vi "CMD_UNLOADSTAMP.vi"(6 "Gantry in":refnum<class "Gantry.lvclass">, 8 "error in (no error)":errorcluster, 10 "Arguments":string[](array[string]), 11 "gScript Interpreter in":refnum<class "gScript Interpreter.lvclass">) -> (0 "error out":errorcluster, 3 "gScript Interpreter out":refnum<class "gScript Interpreter.lvclass">, 4 "Gantry out":refnum<class "Gantry.lvclass">)   [LabVIEW 2017, in "gScript Interpreter.lvclass"]
uses:
  gScript Interpreter.lvclass
  Shared Components/Gantry Class/Gantry.lvclass
  Shared Components/FlexWorktable/FlexWorktable.lvclass
  Shared Components/Vec3d Class/Vec3d.lvclass
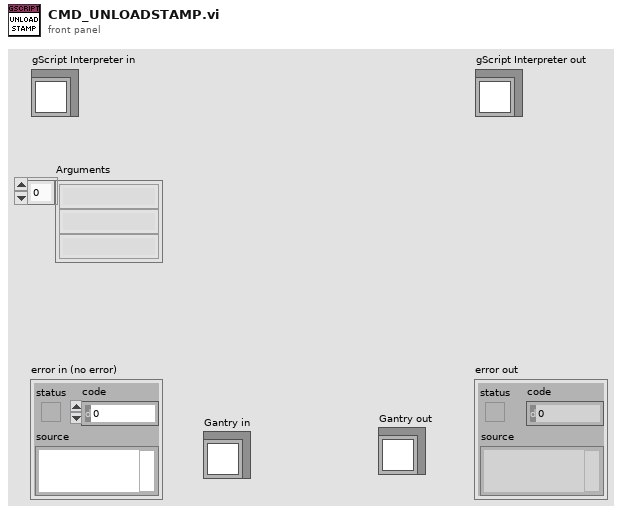
[diagram p1: front panel]
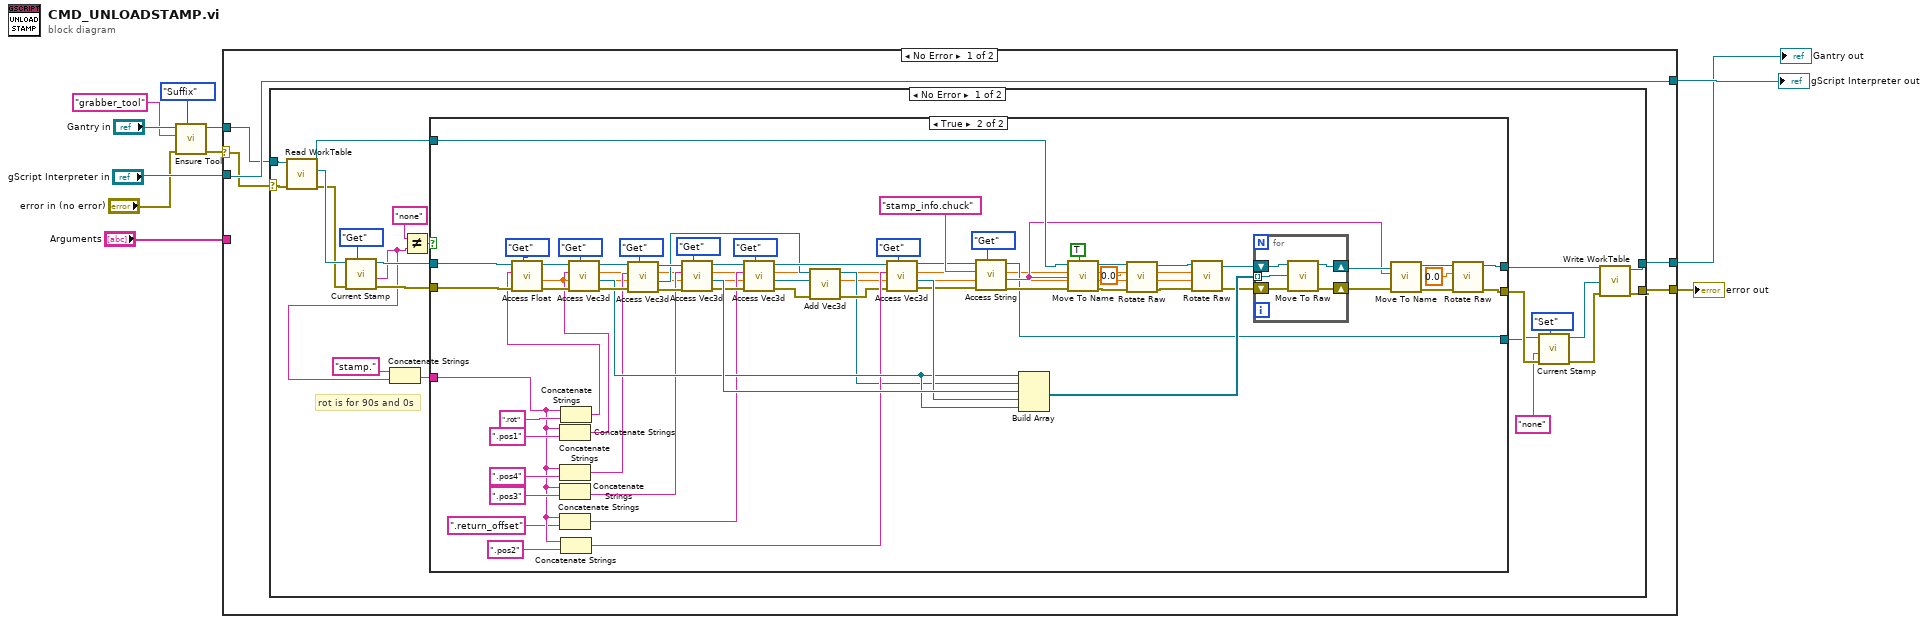
[diagram p0: block diagram]
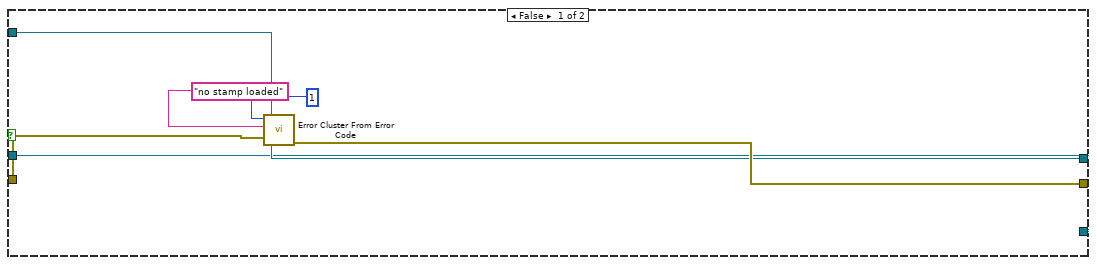
[diagram p2: hidden frame]
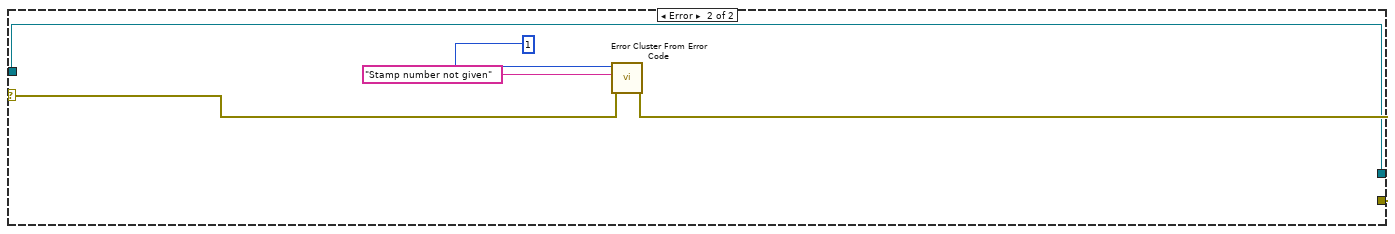
[diagram p3: hidden frame]
diagram:
  n1 = call "Ensure Tool.vi"("Match Type"=enum16{"Full", "Suffix"}."Suffix", "error in (no error)"="error in (no error)", "Tool Name"="grabber_tool", "Gantry in"="Gantry in") -> ("error out"=w3:errorcluster, "Gantry out"=w6:refnum<class "Gantry.lvclass">)  [unwired: 6 in]
  n2 = case shown="No Error" w3 {
    selector: w3 -> [w13 w120]
    tunnel: [w16 w120] -> w11
    tunnel: [w14 w119] -> w9
    tunnel: "gScript Interpreter in" -> [w14 w119]
    tunnel: w6 -> [w12 w118]
    tunnel: [w15 w118] -> w8
    tunnel: "Arguments" -> [_ _]
    frame No Error {
      n3 = case shown="No Error" w13 {
        selector: w13 -> [w38 w114]
        tunnel: [w29 w115] -> w16
        tunnel: w12 -> [w37 w113]
        tunnel: [w28 w113] -> w15
        frame No Error {
          # "rot is for 90s and 0s"
          n4 = call-dynamic "Read WorkTable.vi"("error in"=w38, "Gantry Class in"=w37) -> ("error out"=w23:errorcluster, "Worktable"=w36:refnum<class "FlexWorktable.lvclass">, "Gantry Class out"=w27:refnum<class "Gantry.lvclass">)  [unwired: 7 in]
          n5 = call "Current Stamp.vi"("Get/Set"=enum16{"Get", "Set"}."Get", "error in (no error)"=w23, "FlexWorktable in"=w36) -> ("error out"=w34:errorcluster, "Current Stamp"=w19:string, "FlexWorktable out"=w26:refnum<class "FlexWorktable.lvclass">)  [unwired: 6 in]
          n6 = Concatenate Strings("stamp.", w19) -> (w21:string)
          n7 = Not Equal?(x="none", y=w19) -> (x != y?=w20:bool)
          n8 = case shown="True" w20 {
            tunnel: [w41 w57] -> w30
            tunnel: w34 -> [w42 w91]
            tunnel: w27 -> [w40 w76]
            tunnel: [w40 w56] -> w25
            tunnel: w26 -> [w39 w105]
            tunnel: [w39 w69] -> w24
            tunnel: w21 -> [_ w46]
            frame False {
              n9 = call <vilib>:"Error Cluster From Error Code.vi"("error in (no error)"=w42, "error message (\"\")"="no stamp loaded" ("error message (\"\")"), "error code (0)"=1) -> ("error out"=w41:errorcluster)  [unwired: 6 in]
            }
            frame True {
              n10 = Concatenate Strings(w46, ".pos1" ("string")) -> (w83:string)
              n11 = Concatenate Strings(w46, ".pos4" ("string")) -> (w82:string)
              n12 = Concatenate Strings(w46, ".pos3" ("string")) -> (w81:string)
              n13 = Concatenate Strings(w46, ".return_offset" ("Key")) -> (w62:string)
              n14 = Concatenate Strings(w46, ".rot" ("string")) -> (w79:string)
              n15 = call-dynamic "Access Float.vi"("Get/Set"=enum16{"Get", "Set"}."Get", "error in (no error)"=w91, "Key"=w79, "FlexWorktable in"=w105) -> ("error out"=w107:errorcluster, "Value out"=w52:dbl, "FlexWorktable out"=w106:refnum<class "FlexWorktable.lvclass">)  [unwired: 5 in]
              n16 = Concatenate Strings(w46, ".pos2" ("string")) -> (w80:string)
              n17 = call-dynamic "Access Vec3d.vi"("Get/Set"=enum16{"Get", "Set"}."Get", "error in (no error)"=w107, "Key"=w83, "FlexWorktable in"=w106) -> ("error out"=w104:errorcluster, "Value out"=w89:refnum<class "Vec3d.lvclass">, "FlexWorktable out"=w103:refnum<class "FlexWorktable.lvclass">)  [unwired: 5 in]
              n18 = call-dynamic "Access Vec3d.vi"("Get/Set"=enum16{"Get", "Set"}."Get", "error in (no error)"=w104, "Key"=w82, "FlexWorktable in"=w103) -> ("error out"=w102:errorcluster, "Value out"=w59:refnum<class "Vec3d.lvclass">, "FlexWorktable out"=w101:refnum<class "FlexWorktable.lvclass">)  [unwired: 5 in]
              n19 = call-dynamic "Access Vec3d.vi"("Get/Set"=enum16{"Get", "Set"}."Get", "error in (no error)"=w102, "Key"=w81, "FlexWorktable in"=w101) -> ("error out"=w64:errorcluster, "Value out"=w95:refnum<class "Vec3d.lvclass">, "FlexWorktable out"=w63:refnum<class "FlexWorktable.lvclass">)  [unwired: 5 in]
              n20 = call-dynamic "Access Vec3d.vi"("Get/Set"=enum16{"Get", "Set"}."Get", "error in (no error)"=w64, "Key"=w62, "FlexWorktable in"=w63) -> ("error out"=w65:errorcluster, "Value out"=w66:refnum<class "Vec3d.lvclass">, "FlexWorktable out"=w60:refnum<class "FlexWorktable.lvclass">)  [unwired: 5 in]
              n21 = call-dynamic "Add Vec3d.vi"("error in (no error)"=w65, 10:"Vec3d Class in"=w66, 11:"Vec3d Class in"=w59) -> ("error out"=w61:errorcluster, "Vec3d Class out"=w58:refnum<class "Vec3d.lvclass">)  [unwired: 7 in]
              n22 = call-dynamic "Access Vec3d.vi"("Get/Set"=enum16{"Get", "Set"}."Get", "error in (no error)"=w61, "Key"=w80, "FlexWorktable in"=w60) -> ("error out"=w73:errorcluster, "Value out"=w94:refnum<class "Vec3d.lvclass">, "FlexWorktable out"=w74:refnum<class "FlexWorktable.lvclass">)  [unwired: 5 in]
              n23 = call-dynamic "Access String.vi"("Get/Set"=enum16{"Get", "Set"}."Get", "error in (no error)"=w73, "Key"="stamp_info.chuck", "FlexWorktable in"=w74) -> ("error out"=w75:errorcluster, "Value out"=w70:string, "FlexWorktable out"=w69:refnum<class "FlexWorktable.lvclass">)  [unwired: 5 in]
              n24 = Build Array(w89, w58, w95, w94, w89) -> (w93:refnum<class "Vec3d.lvclass">[])
              n25 = call-dynamic "Move To Name.vi"("Move if Same"=TRUE, "error in"=w75, "Destination"=w70, "Gantry in"=w76) -> ("error out"=w48:errorcluster, "Gantry out"=w51:refnum<class "Gantry.lvclass">)  [unwired: 6 in]
              n26 = call-dynamic "Rotate Raw.vi"("error in"=w48, "position(deg)"=0.0, "Gantry in"=w51) -> ("error out"=w49:errorcluster, "Gantry out"=w50:refnum<class "Gantry.lvclass">)  [unwired: 7 in]
              n27 = call-dynamic "Rotate Raw.vi"("error in"=w49, "speed(deg/s)"=w52, "position(deg)"=w52, "Gantry in"=w50) -> ("error out"=w90:errorcluster, "Gantry out"=w92:refnum<class "Gantry.lvclass">)  [unwired: 6 in]
              n28 = for {
                tunnel: w93 -> [w112] mode=indexing
                shift-right: [w109] -> w71
                shift-left: w90 -> [w108]
                shift-right: [w110] -> w72
                shift-left: w92 -> [w111]
                n29 = call-dynamic "Move To Raw.vi"("error in"=w108, "Destination"=w112, "Gantry in"=w111) -> ("error out"=w109:errorcluster, "Gantry out"=w110:refnum<class "Gantry.lvclass">)  [unwired: 7 in]
              }
              n30 = call-dynamic "Move To Name.vi"("error in"=w71, "Destination"=w70, "Gantry in"=w72) -> ("error out"=w54:errorcluster, "Gantry out"=w55:refnum<class "Gantry.lvclass">)  [unwired: 7 in]
              n31 = call-dynamic "Rotate Raw.vi"("error in"=w54, "position(deg)"=0.0, "Gantry in"=w55) -> ("error out"=w57:errorcluster, "Gantry out"=w56:refnum<class "Gantry.lvclass">)  [unwired: 7 in]
            }
          }
          n32 = call "Current Stamp.vi"("Get/Set"=enum16{"Get", "Set"}."Set", "error in (no error)"=w30, "New Stamp"="none", "FlexWorktable in"=w24) -> ("error out"=w31:errorcluster, "FlexWorktable out"=w32:refnum<class "FlexWorktable.lvclass">)  [unwired: 5 in, 1 out]
          n33 = call-dynamic "Write WorkTable.vi"("error in (no error)"=w31, "FlexWorktable"=w32, "Gantry Class in"=w25) -> ("error out"=w29:errorcluster, "Gantry Class out"=w28:refnum<class "Gantry.lvclass">)  [unwired: 7 in]
        }
        frame Error {
          n34 = call <vilib>:"Error Cluster From Error Code.vi"("error in (no error)"=w114, "error message (\"\")"="Stamp number not given" ("error message (\"\")"), "error code (0)"=1) -> ("error out"=w115:errorcluster)  [unwired: 6 in]
        }
      }
    }
    frame Error {
    }
  }
  "error out" <- w11
  "gScript Interpreter out" <- w9
  "Gantry out" <- w8
